vi "Test Add Event Registration Category.vi"() -> ()   [LabVIEW 2020, in "TEST JKI State Machine API.lvlib"]
uses:
  TEST JKI State Machine API.lvlib
  source/JKI SM/JKI SM.lvclass
panel:
  out "error out":errorcluster
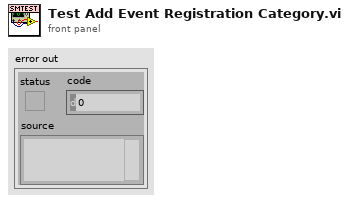
[diagram p1: front panel]
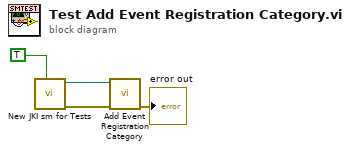
[diagram p0: block diagram]
diagram:
  n1 = call "New JKI sm for Tests.vi"("Open SM FP (for debugging)"=TRUE) -> ("error out"=w2:errorcluster, "JKI SM out"=w3:refnum<class "JKI SM.lvclass">)  [unwired: 9 in]
  n2 = call-dynamic "Add Event Registration Category.vi"("error in (no error)"=w2, "JKI SM in"=w3) -> ("error out"=→"error out":errorcluster)  [unwired: 8 in, 1 out]
